vi "Tosca-Create AI Legend Context Menu.vi"(0 "ListBox in":refnum<vi>, 5 "MenuRef":refnum<k9>, 9 "Coords":T1) -> (8 "discard":bool)   [LabVIEW 2020]
uses:
  <vilib>/Utility/miscctls.llb/LVPoint32TypeDef.ctl
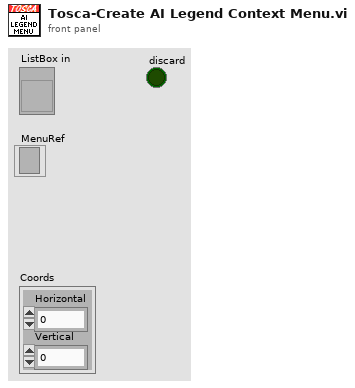
[diagram p1: front panel]
types:
  T1 = typedef "LVPoint32TypeDef.ctl" = cluster{"Horizontal":i32, "Vertical":i32}
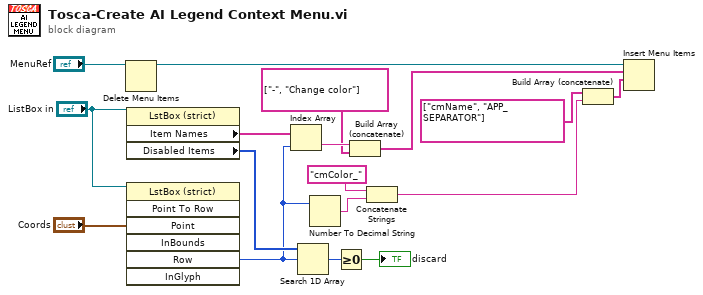
[diagram p0: block diagram]
diagram:
  n1 = Delete Menu Items(9:"MenuRef") -> (3:w14:refnum<k9>)  [unwired: 3 in, 1 out]
  n2 = property on="Property Node" class="LstBox (strict)"(reference="ListBox in") -> ("Item Names"=w4:string[], "Disabled Items"=w11:i32[])  [unwired: 1 in, 2 out]
  n3 = invoke on="Invoke Node" class="LstBox (strict)" method="Point To Row"(reference="ListBox in", "Point"="Coords") -> ("Row"=w2:i32)  [unwired: 5 in, 6 out]
  n4 = Index Array(array=w4, index=w2) -> (element=w13:string)
  n5 = Search 1D Array(1D array=w11, element=w2) -> (index of element=w10:i32)  [unwired: 1 in]
  n6 = Number To Decimal String(number=w2) -> (decimal integer string=w1:string)  [unwired: 1 in]
  n7 = Greater Or Equal To 0?(x=w10) -> (x >= 0?=→"discard":bool)
  n8 = Build Array (concatenate)(w13, string[] ["-", "Change color"] ("item tags")) -> (w12:string[])
  n9 = Concatenate Strings("cmColor_" ("string"), w1) -> (w3:string)
  n10 = Build Array (concatenate)(string[] ["cmName", "APP_SEPARATOR"] ("item tags"), w3) -> (w6:string[])
  n11 = Insert Menu Items(7:w6, 8:w12, 9:w14) -> ()  [unwired: 3 in, 3 out]
